vi "Read Filter.vi"(8 "error in":errorcluster) -> (0 "error out":errorcluster)   [LabVIEW 2015]
uses:
  Controls/Flags.ctl
  <vilib>/DAQmx/read.llb/DAQmx Read (Digital 1D Bool NChan 1Samp 1Line).vi
  <vilib>/DAQmx/miscellaneous.llb/DAQmx Fill In Error Info.vi
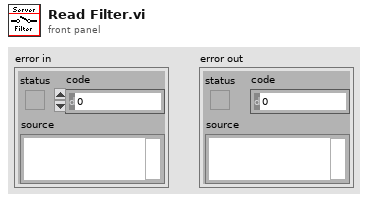
[diagram p1: front panel]
types:
  T1 = typedef "Flags.ctl" = enum8{"Autospeaker", "Link cycles", "Autofilter", "O3 Cal", "Filter Position"}
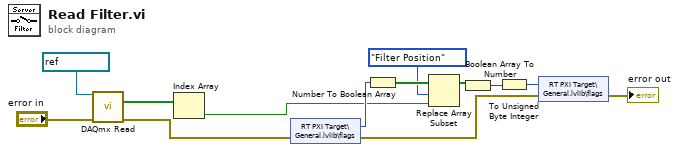
[diagram p0: block diagram]
diagram:
  n1 = call-poly <vilib>:"DAQmx Read.vi"("task/channels in"=refnum<k21> "Filter In", "error in"="error in") -> ("data"=w12:bool[], "error out"=w3:errorcluster)  [unwired: 11 in, 1 out]
  n2 = Index Array(array=w12) -> (element=w1:bool)  [unwired: 1 in]
  n3 = shared-variable "RT PXI Target\\General.lvlib\\flags"(error in=w3) -> (w9:u8, error out=w10:errorcluster)
  n4 = Number To Boolean Array(number=w9) -> (Boolean array=w8:bool[])
  n5 = Replace Array Subset(array=w8, new element=w1, index=Flags."Filter Position" ("Flags")) -> (w7:bool[])
  n6 = Boolean Array To Number(Boolean array=w7) -> (number=w6:u32)
  n7 = To Unsigned Byte Integer(number=w6) -> (unsigned 8bit integer=w5:u8)
  n8 = shared-variable "RT PXI Target\\General.lvlib\\flags"(w5, error in=w10) -> (error out=→"error out":errorcluster)
